vi "Stage Launcher.vi"(9 "Sub Panel":refnum<vi>, 11 "Panel Actor In":refnum<class "Main.lvclass">) -> (2 "Nested Actor's Enqueuer":refnum<class "Message Enqueuer.lvclass">, 3 "Panel Actor Out":refnum<class "Main.lvclass">)   [LabVIEW 2018, in "Stage Actor.lvlib" / "Stage.lvclass"]
uses:
  Stage.lvclass
  ADM/ADM/Main.lvclass
  C:/Program Files (x86)/National Instruments/LabVIEW 2018/vi.lib/MGI/Panel Manager/Panel Actor/Panel Actor/Panel Actor.lvclass
  <vilib>/ActorFramework/Message Enqueuer/Message Enqueuer.lvclass
  Stage.lvclass/Stage.ctl
  <vilib>/MGI/Panel Manager/Panel/Panel/Subpanel/Subpanel.lvclass
  C:/Program Files (x86)/National Instruments/LabVIEW 2018/vi.lib/MGI/Panel Manager/Panel/Panel/Panel.lvclass
  <vilib>/MGI/Panel Manager/Panel/Panel/Subpanel/Subpanel.vi
  <vilib>/MGI/Panel Manager/Panel/Panel.lvlib
  <vilib>/MGI/Panel Manager/Panel Actor/Panel Actor/Panel Actor.lvclass
  <instrlib>/Zaber A Series/Zaber A Series.lvlib
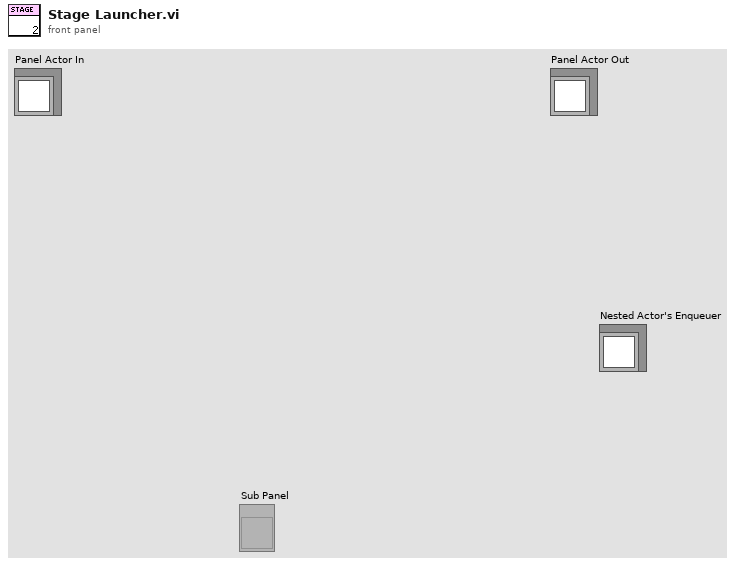
[diagram p1: front panel]
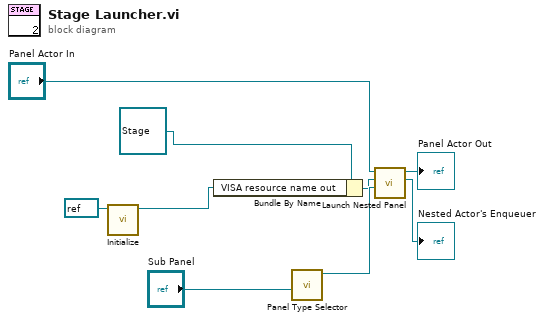
[diagram p0: block diagram]
diagram:
  n1 = call <instrlib>:"Initialize.vi"("VISA resource name"=refnum<visa-resource-name> refnum) -> ("VISA resource name out"=w2:refnum<visa-resource-name>)  [unwired: 9 in, 1 out]
  n2 = Bundle By Name(cluster=refnum<class "Stage.lvclass"> refnum ("Stage Actor.lvlib:Stage.lvclass"), "VISA resource name out"=w2) -> (w6:refnum<class "Stage.lvclass">)
  n3 = call-poly <vilib>:"Panel Type Selector.vi"("Sub Panel"="Sub Panel") -> ("Subpanel Out"=w7:refnum<class "Subpanel.lvclass">)  [unwired: 9 in, 1 out]
  n4 = call <vilib>:"Launch Nested Panel.vi"("Panel"=w7, "Nested Panel Actor"=w6, "Panel Actor in"="Panel Actor In") -> ("Nested Actor's Enqueuer"=→"Nested Actor's Enqueuer":refnum<class "Message Enqueuer.lvclass">, "Panel Actor out"=→"Panel Actor Out":refnum<class "Main.lvclass">)  [unwired: 5 in, 2 out]
